vi "Arguments - Safe Arguments if it contains key words of CSM.vi"() -> ()   [LabVIEW 2014]
uses:
  user.lib/_NEVSTOP/Communicable State Machine(CSM)/AdvanceAPI/CSM - Keywords.vi
  user.lib/_NEVSTOP/Communicable State Machine(CSM)/Communicable State Machine.lvlib
panel:
  in  "Argurment String 3":string="https://github.com/NEVSTOP-LAB/Communicable-State-Machine"
  out "Safe Argurment String 3":string="https:%2F%2Fgithub.com/NEVSTOP-LAB/Communicable-State-Machine"
  out "Safe Argurment String 2":string="c:\\abc\\def.txt"
  in  "Argurment String 2":string="c:\\abc\\def.txt"
  out "Safe Argurment String":string="eaasdf%2D%3Efqwvrf%2D%26#%0Adddd\\\\\\\\\\not comments%0A%2F%2Fadcd\\\\de/assfd%0A%2C %5B%3B%5D%0A%2D%40asdfvq%3C%2D1234"
  out "Origin Argurment String":string="eaasdf->fqwvrf-&#\ndddd\\\\\\\\\\not comments\n//adcd\\\\de/assfd\n, [;]\n-@asdfvq<-1234"
  in  "Argurment String":string="eaasdf->fqwvrf-&#\ndddd\\\\\\\\\\not comments\n//adcd\\\\de/assfd\n, [;]\n-@asdfvq<-1234"
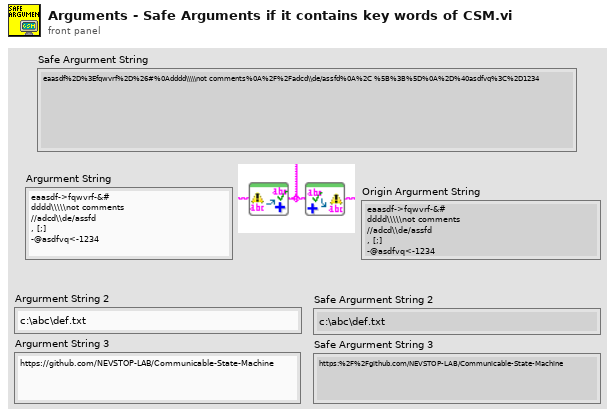
[diagram p1: front panel]
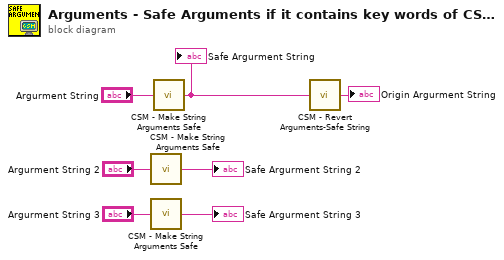
[diagram p0: block diagram]
diagram:
  n1 = call "CSM - Make String Arguments Safe.vi"("Argurment String"="Argurment String 2") -> ("Safe Argurment String"=→"Safe Argurment String 2":string)  [unwired: 8 in]
  n2 = call "CSM - Make String Arguments Safe.vi"("Argurment String"="Argurment String 3") -> ("Safe Argurment String"=→"Safe Argurment String 3":string)  [unwired: 8 in]
  n3 = call "CSM - Make String Arguments Safe.vi"("Argurment String"="Argurment String") -> ("Safe Argurment String"=w6:string)  [unwired: 8 in]
  "Safe Argurment String" <- w6
  n4 = call "CSM - Revert Arguments-Safe String.vi"("Safe Argurment String"=w6) -> ("Origin Argurment String"=→"Origin Argurment String":string)  [unwired: 8 in]
